vi "saveLogEntry.vi"(8 "error in (no error)":errorcluster, 11 "Logger in":refnum<class "StiffnessLog.lvclass">) -> (0 "error out":errorcluster, 3 "Logger out":refnum<class "StiffnessLog.lvclass">)   [LabVIEW 2013, in "StiffnessLog.lvclass"]
uses:
  StiffnessLog.lvclass
  StiffnessLog.lvclass/StiffnessLog.ctl
  <userlib>/Common/Log/Log/Log.lvclass/Log.ctl
  <userlib>/Common/Log/Log/Log.lvclass
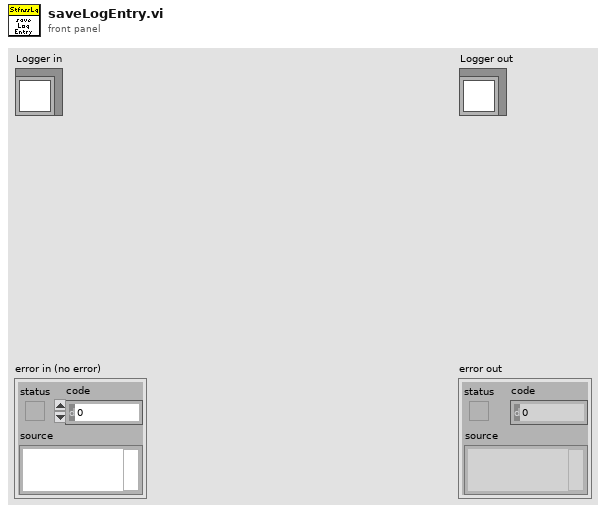
[diagram p1: front panel]
types:
  T1 = typedef "M2AADTTypedefs.lvlib/StiffnessData.ctl" = cluster{"Constrained Displacement":dbl[unit], "Stiffness":dbl[unit]}
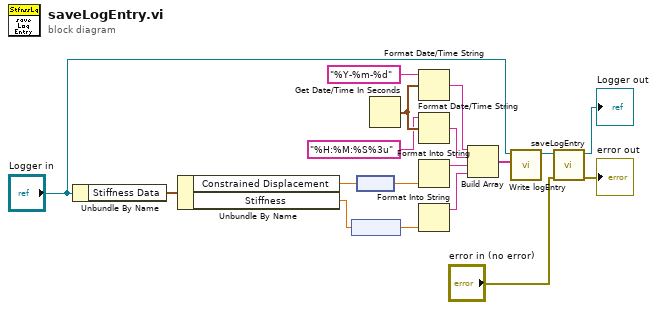
[diagram p0: block diagram]
diagram:
  n1 = Unbundle By Name("Logger in") -> ("Stiffness Data"=w7:T1)
  n2 = Unbundle By Name(w7) -> ("Constrained Displacement"=w6:dbl[unit], "Stiffness"=w5:dbl[unit])
  n3 = node(w5) -> (w4:dbl)
  n4 = node(w6) -> (w3:dbl)
  n5 = Get Date/Time In Seconds() -> (seconds since 1Jan1904=w17:timestamp)
  n6 = Format Date/Time String(time format string (%c)="%Y-%m-%d" ("format string"), seconds (now)=w17) -> (date/time string=w14:string)  [unwired: 1 in]
  n7 = Format Date/Time String(time format string (%c)="%H:%M:%S%3u", seconds (now)=w17) -> (date/time string=w15:string)  [unwired: 1 in]
  n8 = Format Into String(w3) -> (resulting string=w2:string)  [unwired: 3 in, 1 out]
  n9 = Format Into String(w4) -> (resulting string=w1:string)  [unwired: 3 in, 1 out]
  n10 = Build Array(w14, w15, w2, w1) -> (w11:string[])
  n11 = call <userlib>:"Write logEntry.vi"("logEntry"=w11, "Logger in"="Logger in") -> ("Logger out"=w12:refnum<class "StiffnessLog.lvclass">)  [unwired: 9 in]
  n12 = call-parent "saveLogEntry.vi"("error in (no error)"="error in (no error)", "Logger in"=w12) -> ("error out"=→"error out":errorcluster, "Logger out"=→"Logger out":refnum<class "StiffnessLog.lvclass">)  [unwired: 8 in]
